vi "Get Measure Configuration List Size.vi"(8 "error in (no error)":errorcluster, 10 "Configuration List Name":string="myList", 11 "VISA resource name":refnum<visa-resource-name>) -> (0 "error out":errorcluster, 2 "Measure Configuration List Size":i32, 3 "VISA resource name out":refnum<visa-resource-name>)   [LabVIEW 2020, in "Keithley 2450.lvlib"]
doc: "This gets the Measure configuration list Size"
uses:
  Keithley 2450.lvlib
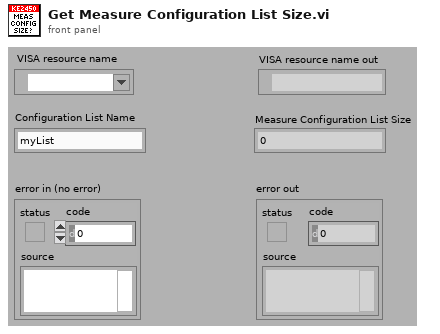
[diagram p1: front panel]
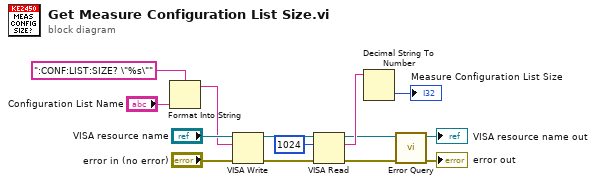
[diagram p0: block diagram]
diagram:
  n1 = Format Into String(format string=":CONF:LIST:SIZE? \"%s\"", "Configuration List Name") -> (resulting string=w2:string)  [unwired: 2 in, 1 out]
  n2 = VISA Write(VISA resource name="VISA resource name", write buffer=w2, error in (no error)="error in (no error)") -> (VISA resource name out=w13:refnum<visa-resource-name>, error out=w14:errorcluster)  [unwired: 1 out]
  n3 = VISA Read(VISA resource name=w13, byte count=u32 1024, error in (no error)=w14) -> (VISA resource name out=w6:refnum<visa-resource-name>, read buffer=w7:string, error out=w5:errorcluster)  [unwired: 1 out]
  n4 = Decimal String To Number(string=w7) -> (number=→"Measure Configuration List Size":i32)  [unwired: 2 in, 1 out]
  n5 = call "Error Query.vi"("error in (no error)"=w5, "VISA resource name"=w6) -> ("error out"=→"error out":errorcluster, "VISA resource name out"=→"VISA resource name out":refnum<visa-resource-name>)  [unwired: 8 out]
